vi "gl_Windows Ctrl refs.vi"() -> ()   [LabVIEW 2013]
uses:
  Subpanel Windows/SubVIs/Typedefs/Live window-ctrl refs.ctl
  Typedefs/Channel Selector.ctl
  Typedefs/Image display ref.ctl
panel:
  out "Refresh live img UI":bool
  in  "Linked sliders":bool
  out "Sliders distance (right)":i16
  out "Sliders distance (left)":i16
  in  "Slider distance locked (right)":bool
  in  "Slider distance locked (left)":bool
  in  "Live img window ctrl refs":T1
  # "This is set TRUE when a user or user profile has been switched."
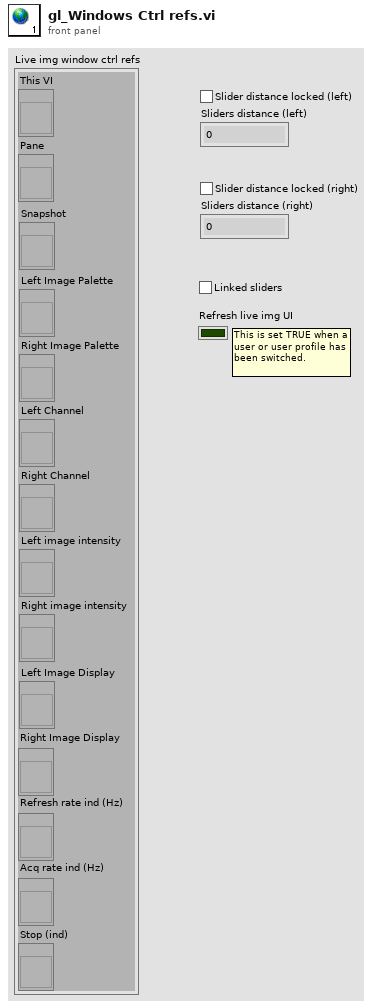
[diagram p1: front panel]
types:
  T1 = typedef "Live window-ctrl refs.ctl" = cluster{"This VI":refnum<vi>, "Pane":refnum<vi>, "Snapshot":refnum<vi>, "Left Image Palette":refnum<vi>, "Right Image Palette":refnum<vi>, "Left Channel":refnum<vi>, "Right Channel":refnum<vi>, "Left image intensity":refnum<vi>, "Right image intensity":refnum<vi>, "Left Image Display":T2, "Right Image Display":T2, "Refresh rate ind (Hz)":refnum<vi>, "Acq rate ind (Hz)":refnum<vi>, "Stop (ind)":refnum<vi>}
  T2 = typedef "Image display ref.ctl" = refnum<vi>
diagram:
